vi "LEP_RV_ClearDebugSymbol.vi"(8 "error in":errorcluster) -> (0 "error out":errorcluster)   [LabVIEW 2011]
uses:
  <vilib>/Platform/EmbProject/Plugins/utilities/LEP_Utilities_GetSetProjectData_String.vi
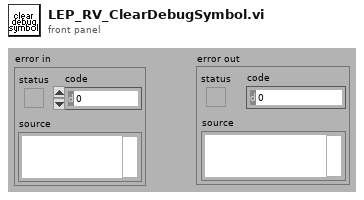
[diagram p1: front panel]
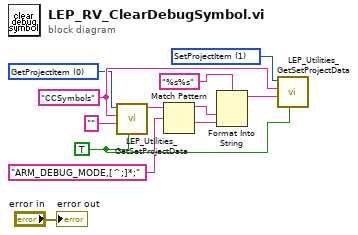
[diagram p0: block diagram]
diagram:
  w10 = u16 0 items=["GetProjectItem", "SetProjectItem"] ("Command")
  w12 = u16 1 items=["GetProjectItem", "SetProjectItem"] ("Command")
  w8 = TRUE ("access target data (F)")
  w11 = "CCSymbols" ("Name")
  n1 = call-poly <vilib>:"LEP_Utilities_GetSetProjectData.vi"("access target data (F)"=w8, "data in"="" ("Name"), "ItemName"=w11, "Command"=w10) -> ("data out"=w7:string)  [unwired: 1 in, 6 out]
  n2 = Match Pattern(string=w7, regular expression="ARM_DEBUG_MODE,[^;]*;" ("format string")) -> (before substring=w4:string, after substring=w3:string)  [unwired: 1 in, 2 out]
  n3 = Format Into String(format string="%s%s", w4, w3) -> (resulting string=w2:string)  [unwired: 2 in, 1 out]
  n4 = call-poly <vilib>:"LEP_Utilities_GetSetProjectData.vi"("access target data (F)"=w8, "data in"=w2, "ItemName"=w11, "Command"=w12) -> ()  [unwired: 1 in, 7 out]
  "error out" <- "error in"
